vi "Remove_Current_Active_Car_Call.vi"(8 "error in (no error)":errorcluster, 9 "Car Calls in":T1, 10 "Elevator in":T2, 11 "Elevator Fleet in":T9) -> (0 "error out":errorcluster, 1 "Car Calls out":T1, 2 "Elevator out":T2, 3 "Elevator Fleet out":T9)   [LabVIEW 2026]
uses:
  Controls/Elevator_Status.ctl
  Controls/Door_Status_Enum.ctl
  Controls/Occupy_Status.ctl
  Controls/Floor_Status.ctl
  Controls/Motion_Status_Enum.ctl
  Controls/Car_Calls_Status.ctl
  Controls/Hall_Calls_Status.ctl
  Controls/Elevator_Fleet.ctl
  Controls/Car_Calls.ctl
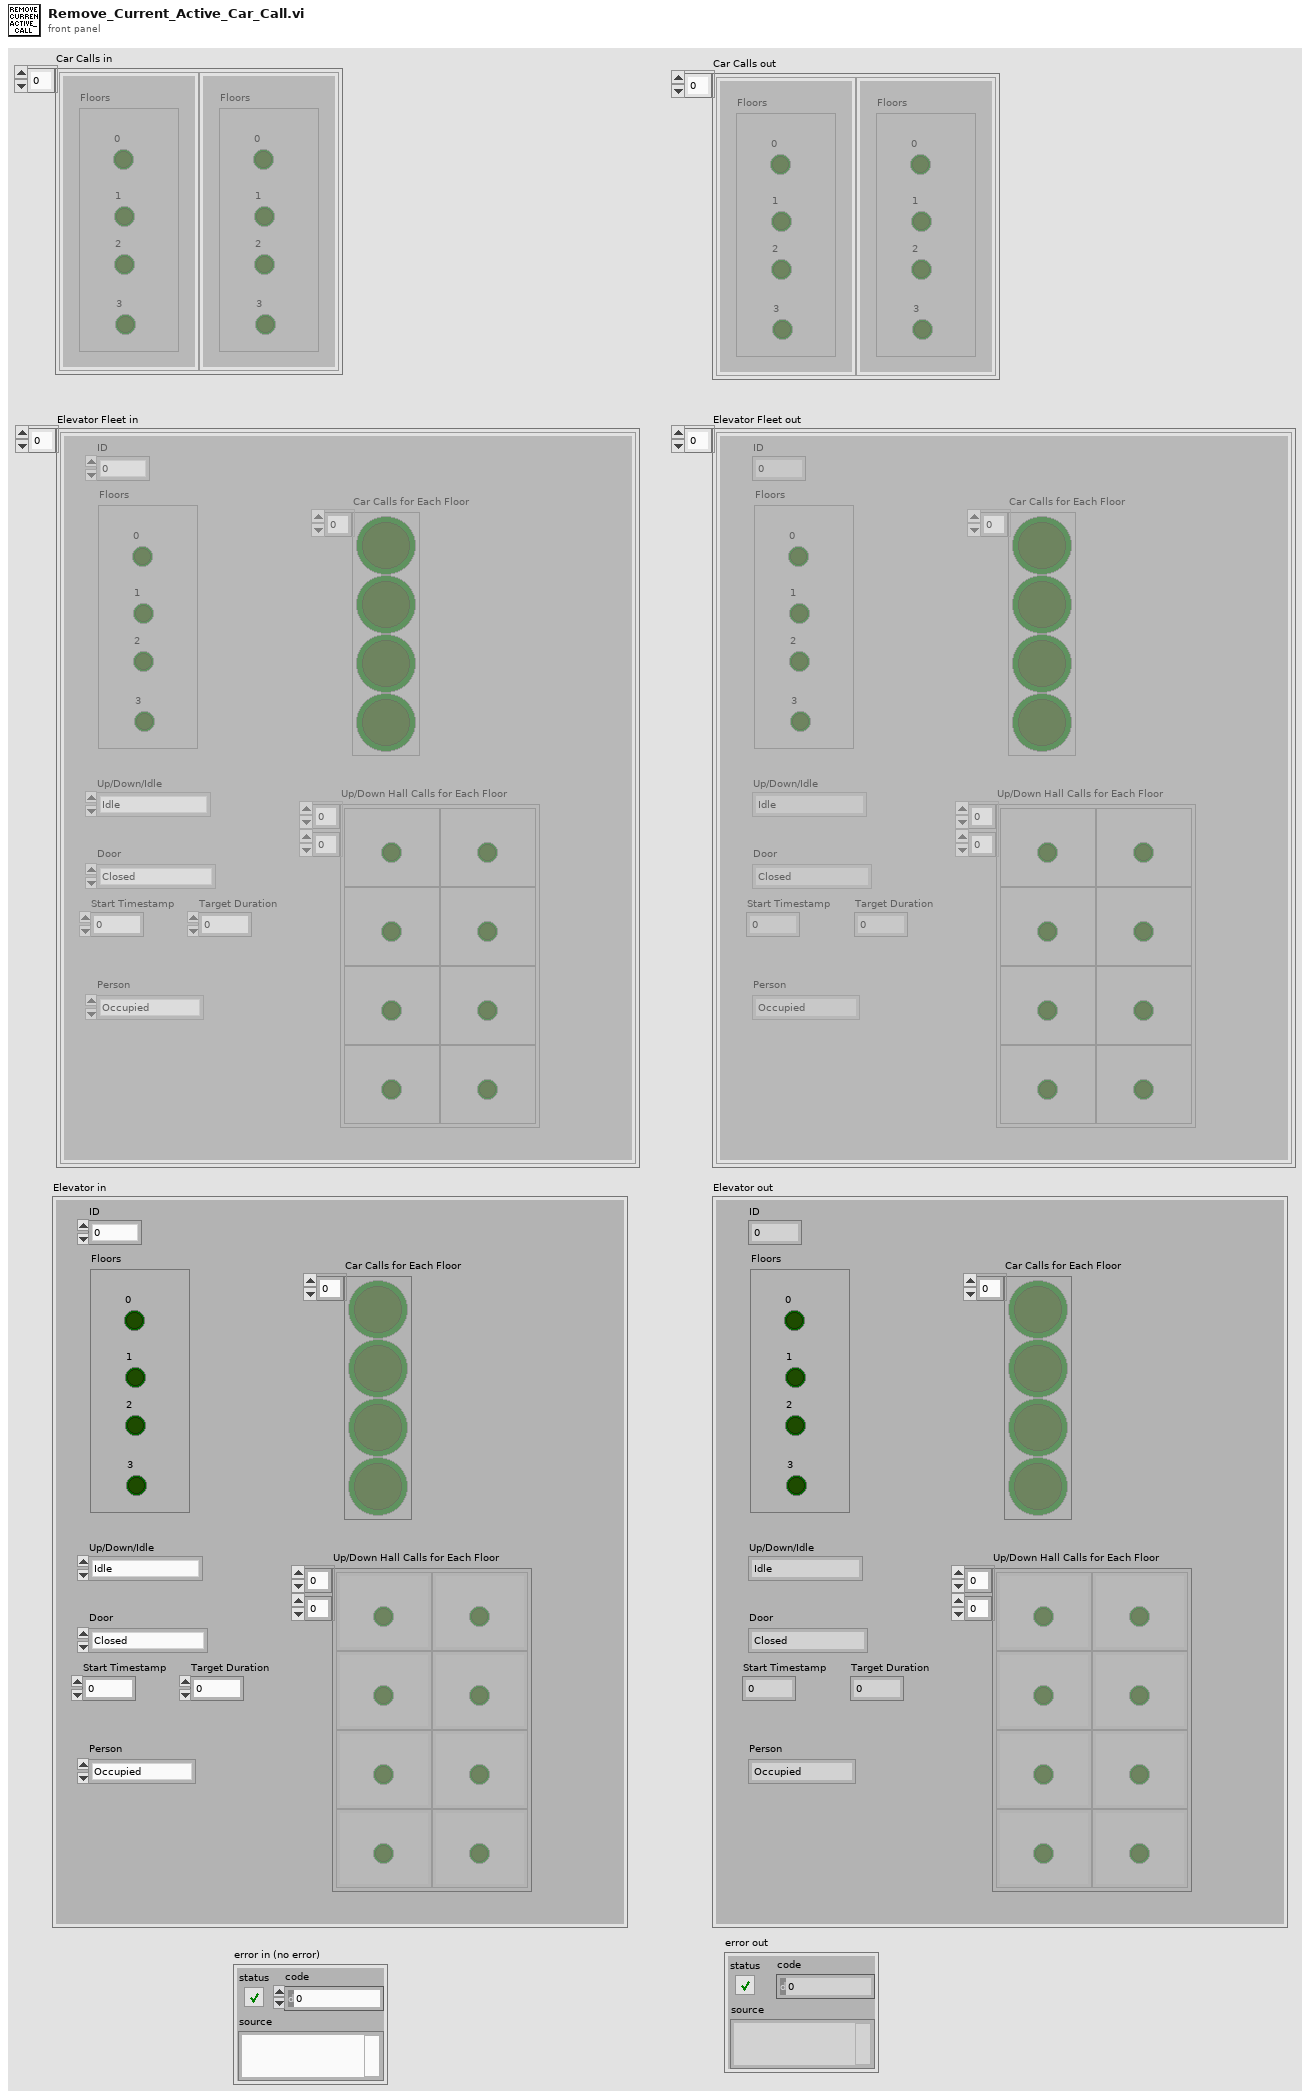
[diagram p1: front panel]
types:
  T1 = typedef "Car_Calls.ctl" = cluster{"Floors":cluster{"0":bool, "1":bool, "2":bool, "3":bool}}[]
  T2 = typedef "Elevator_Status.ctl" = cluster{"Door":T3, "Person":T4, "Floors":T5, "Up/Down/Idle":T6, "Car Calls for Each Floor":T7, "Up/Down Hall Calls for Each Floor":T8, "ID":i32, "Start Timestamp":u32, "Target Duration":dbl}
  T3 = typedef "Door_Status_Enum.ctl" = enum16{"Closed", "Open", "Opening", "Closing"}
  T4 = typedef "Occupy_Status.ctl" = enum16{"Occupied", "Empty"}
  T5 = typedef "Floor_Status.ctl" = cluster{"0":bool, "1":bool, "2":bool, "3":bool}
  T6 = typedef "Motion_Status_Enum.ctl" = enum16{"Idle", "Up", "Down"}
  T7 = typedef "Car_Calls_Status.ctl" = bool[]
  T8 = typedef "Hall_Calls_Status.ctl" = cluster{bool}[][]
  T9 = typedef "Elevator_Fleet.ctl" = T2[]
  T10 = enum16{"Check for Any Floor - Car Call", "Check for Specific Floor - Car Call", "Check for Any Floor - Hall Call", "Check for Specific Floor - Hall Call"}
  T11 = cluster{"Floors":cluster{"0":bool, "1":bool, "2":bool, "3":bool}}
  T12 = cluster{"Floors[0]":bool, "Floors[1]":bool, "Floors[2]":bool, "Floors[3]":bool}
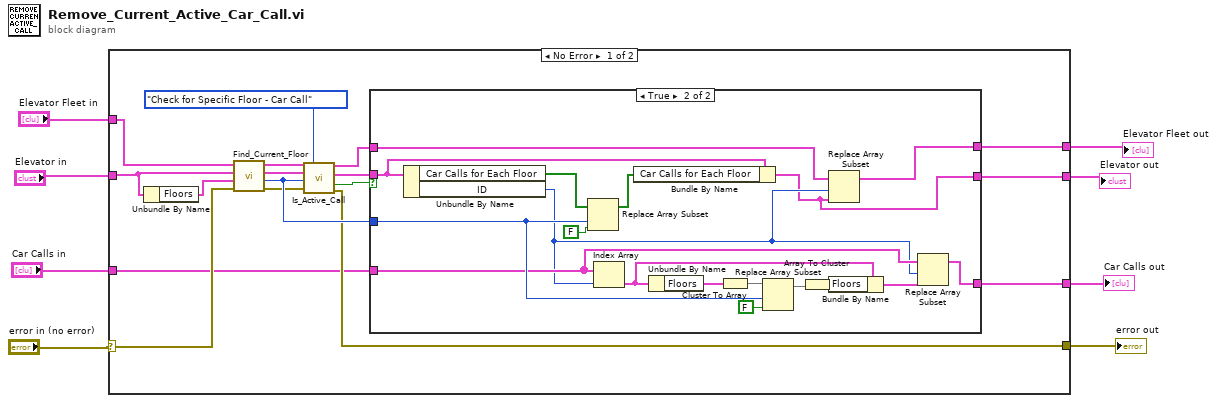
[diagram p0: block diagram]
diagram:
  n1 = case shown="No Error" "error in (no error)" {
    selector: "error in (no error)" -> [w18 w50]
    tunnel: "Elevator in" -> [w15 w49]
    tunnel: "Elevator Fleet in" -> [w21 w48]
    tunnel: [w12 w49] -> w5
    tunnel: [w16 w50] -> w4
    tunnel: [w13 w48] -> w3
    tunnel: "Car Calls in" -> [w10 w47]
    tunnel: [w9 w47] -> w1
    frame No Error {
      n2 = Unbundle By Name(w15) -> ("Floors"=w19:T5)
      n3 = call "Find_Current_Floor.vi"("error in (no error)"=w18, "Floors"=w19, "Elevator Status in"=w15, "Elevator Fleet in"=w21) -> ("error out"=w17:errorcluster, "Current Floor"=w22:i32, "Elevator Status out"=w25:T2, "Elevator Fleet out"=w20:T9)  [unwired: 4 in]
      n4 = call "Is_Active_Call.vi"("Elevator Fleet in"=w20, "Enum"=T10."Check for Specific Floor - Car Call", "Elevator in"=w25, "Floor"=w22, "error in (no error)"=w17) -> ("Elevator Fleet out"=w14:T9, "Elevator out"=w23:T2, "Active Call?"=w24:bool, "error out"=w16:errorcluster)  [unwired: 6 in, 1 out]
      n5 = case shown="True" w24 {
        tunnel: w23 -> [w27 w44]
        tunnel: w22 -> [_ w38]
        tunnel: [w28 w41] -> w13
        tunnel: w14 -> [w28 w42]
        tunnel: [w27 w29] -> w12
        tunnel: w10 -> [w26 w32]
        tunnel: [w26 w30] -> w9
        frame False {
        }
        frame True {
          n6 = Unbundle By Name(w44) -> ("Car Calls for Each Floor"=w46:T7, "ID"=w31:i32)
          n7 = Replace Array Subset(array=w46, new element=FALSE ("new element/subarray"), index=w38) -> (w43:T7)
          n8 = Index Array(array=w32, index=w31) -> (element=w34:T11)
          n9 = Bundle By Name(cluster=w44, "Car Calls for Each Floor"=w43) -> (w29:T2)
          n10 = Unbundle By Name(w34) -> ("Floors"=w40:cluster{"0":bool, "1":bool, "2":bool, "3":bool})
          n11 = Cluster To Array(cluster=w40) -> (array=w39:bool[])
          n12 = Replace Array Subset(array=w39, new element=FALSE ("new element/subarray"), index=w38) -> (w36:bool[])
          n13 = Array To Cluster(array=w36) -> (cluster=w35:T12)
          n14 = Replace Array Subset(array=w42, new element=w29, index=w31) -> (w41:T9)
          n15 = Bundle By Name(cluster=w34, "Floors"=w35) -> (w33:T11)
          n16 = Replace Array Subset(array=w32, new element=w33, index=w31) -> (w30:T1)
        }
      }
    }
    frame Error {
    }
  }
  "Elevator Fleet out" <- w3
  "Elevator out" <- w5
  "error out" <- w4
  "Car Calls out" <- w1
